vi "Construct String Expression Formatter.vi"(6 "Remove LineFeeds?(F)":bool, 7 "Append EOL?":bool=TRUE, 8 "error in (no error)":errorcluster, 11 "Format Specifier":string) -> (0 "error out":errorcluster, 3 "String Expression Format out":refnum<class "String Expression Format.lvclass">)   [LabVIEW 2019, in "String Expression Format.lvclass"]
doc: "Construct a string expression formatter - a string expression can be used to define the format of a sink's log entries. Use the keys [EVT], [TIME], [ID], and [LVL] to apply formatting to the event, time, source, and level fields of the event. Any text before the key (and after a prior key) will be used in a 'format into string' function for that particular event field. See format into string function details for valid format specifiers.\n\nUse the error IO of this method to verify your format string before injecting into a sink."
uses:
  <vilib>/gpm_packages/@cs/event-logger/Source/String Formats/String Expression Format/String Expression Format.lvclass
  <vilib>/gpm_packages/@cs/event-logger/Source/String Formats/String Expression Format/String Expression Format.lvclass/String Expression Format.ctl
  <vilib>/dlg_ctls.llb/Space Constant.vi
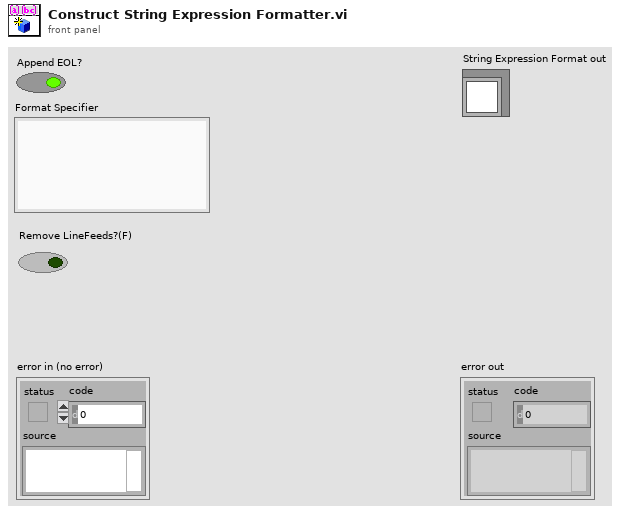
[diagram p1: front panel]
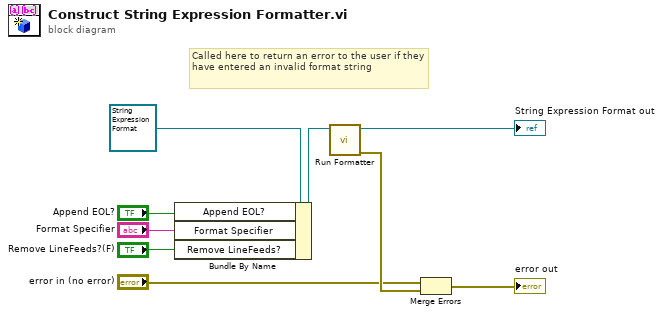
[diagram p0: block diagram]
diagram:
  # "Called here to return an error to the user if they have entered an invalid format string"
  n1 = Bundle By Name(cluster=refnum<class "String Expression Format.lvclass"> refnum ("String Expression Format in"), "Append EOL?"="Append EOL?", "Format Specifier"="Format Specifier", "Remove LineFeeds?"="Remove LineFeeds?(F)") -> (w6:refnum<class "String Expression Format.lvclass">)
  n2 = call <vilib>:"Run Formatter.vi"("String Expression Format in"=w6) -> ("error IO"=w4:errorcluster, "String Expression Format out"=→"String Expression Format out":refnum<class "String Expression Format.lvclass">)  [unwired: 8 in, 1 out]
  n3 = Merge Errors("error in (no error)", w4) -> (→"error out":errorcluster)
